vi "NI-Embedded CAN for RIO subVI - CAN Frame to Table1.vi"(6 "ramki":bool, 7 "Hexadecimal?":bool, 8 "error in (no error)":errorcluster, 9 "timestamp":timestamp, 10 "CAN frame":T1 {"type" items=["CAN Data", "CAN Remote"]; "identifier" format="%.0x"}, 11 "Input Array":string[][](array[string])) -> (0 "appended array":string[](array[string]), 1 "okres 1000":dbl, 3 "Output Array":string[][](array[string]), 4 "ilosc mesagy":dbl, 5 "okres 100":dbl)   [LabVIEW 2015]
doc: "This example shows how to put a CAN transceiver to sleep on RIO Embedded CAN devices."
uses:
  <vilib>/RioEmbeddedCAN/RioEmbeddedCAN.llb/CANFrameControl.ctl
panel:
  out "subarray 2":string[](array[string])
  out "subarray":string[](array[string])
  in  "Array":T1[](array[typedef]) {"type" items=["CAN Data", "CAN Remote"]; "identifier" format="%.0x"}
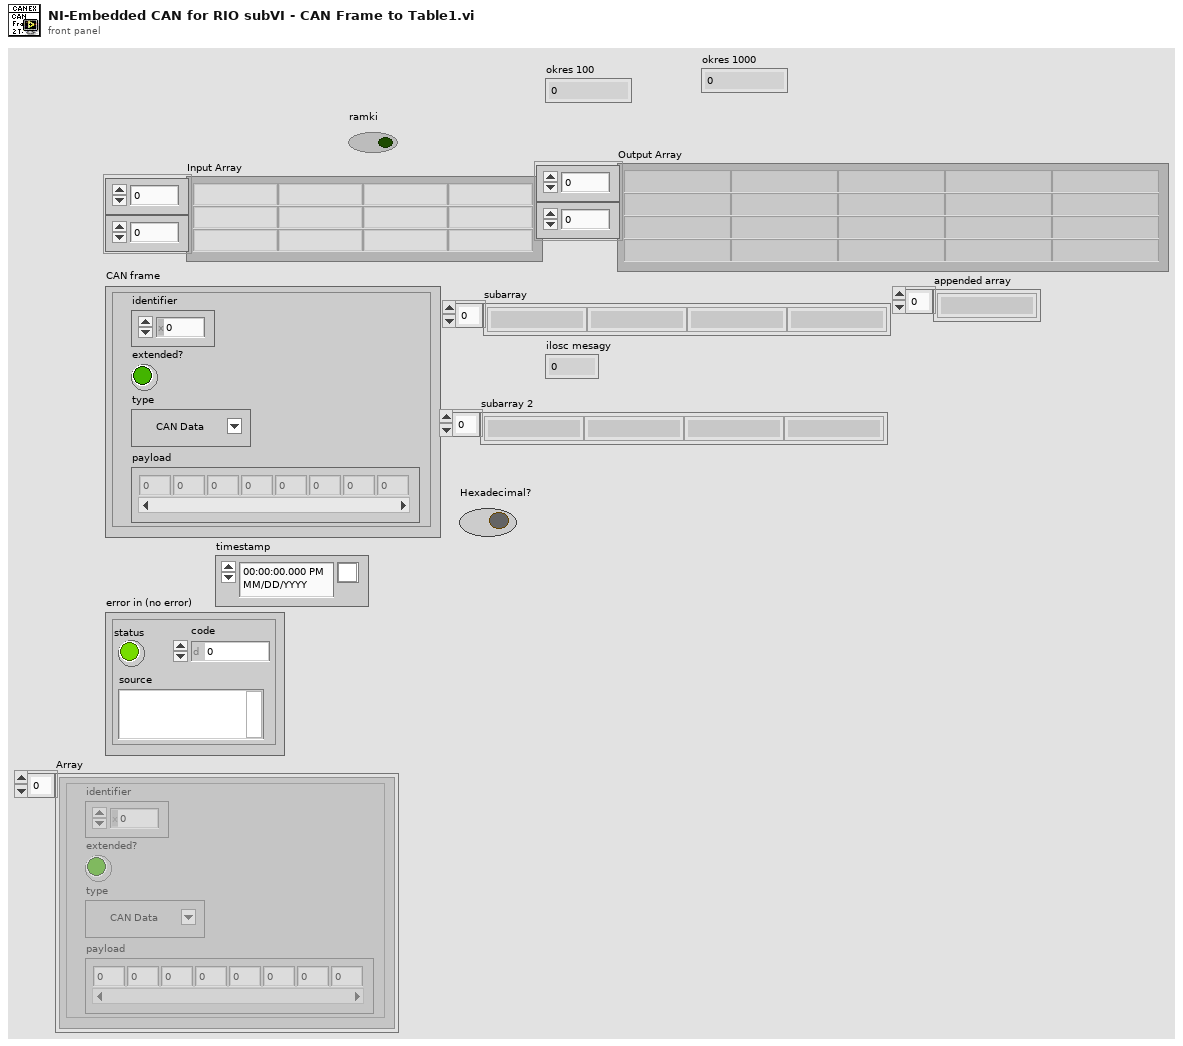
[diagram p1: front panel]
types:
  T1 = typedef "CANFrameControl.ctl" = cluster{"identifier":u32, "extended?":bool, "type":u8, "payload":u8[]}
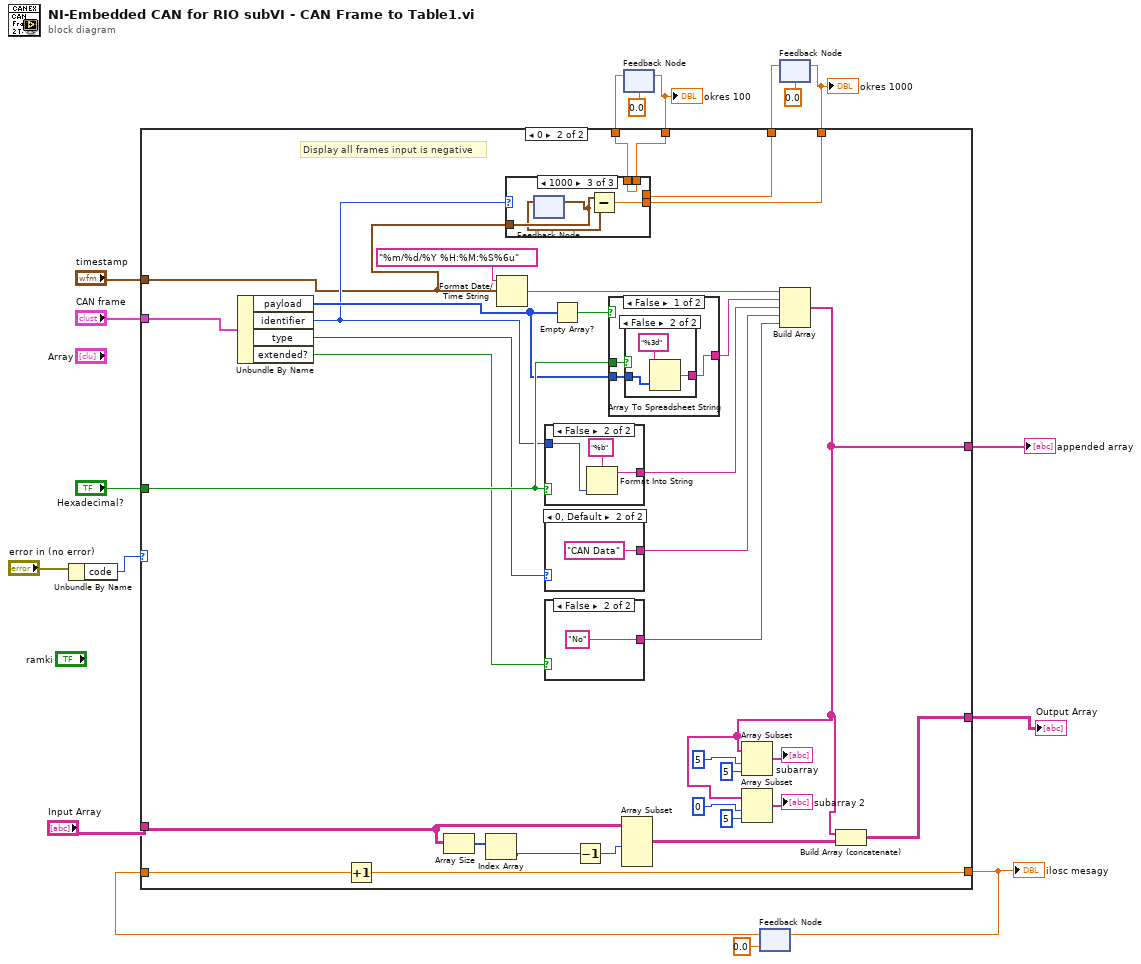
[diagram p0: block diagram]
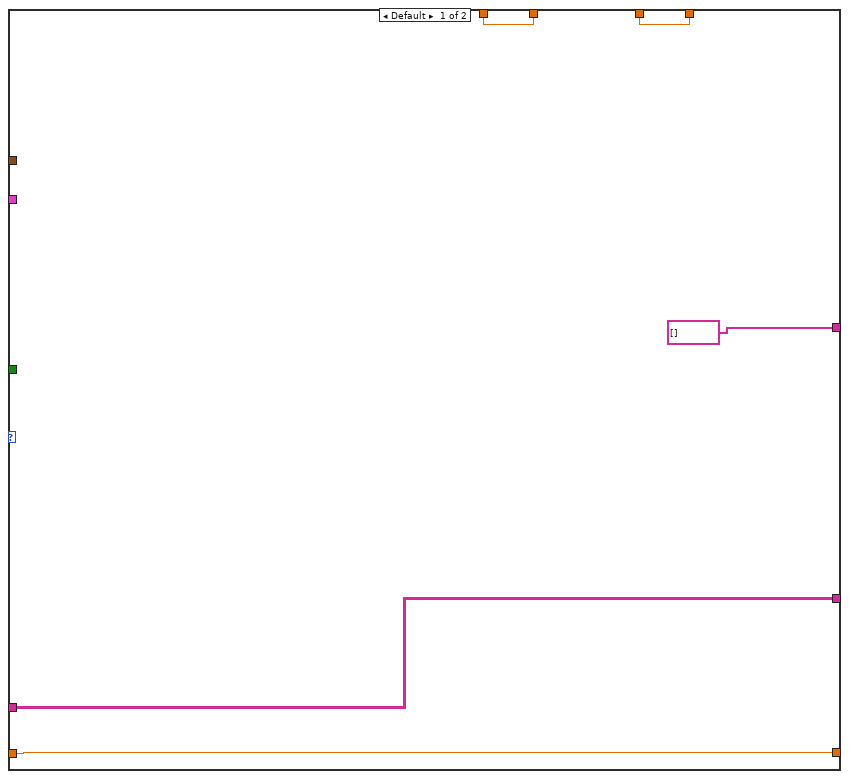
[diagram p2: hidden frame]
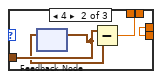
[diagram p4: hidden frame]
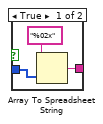
[diagram p5: hidden frame]
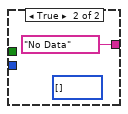
[diagram p6: hidden frame]
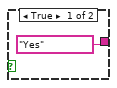
[diagram p7: hidden frame]
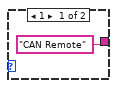
[diagram p8: hidden frame]
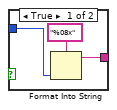
[diagram p9: hidden frame]
diagram:
  n1 = Unbundle By Name("error in (no error)") -> ("code"=w6:i32)
  n2 = feedback #1(0.0) -> (w4:dbl)
  n3 = feedback #2(0.0) -> (w10:dbl)
  n4 = feedback #3(0.0) -> (w3:dbl)
  n5 = case shown="0" w6 {
    tunnel: "Input Array" -> [w22 w54]
    tunnel: [w22 w53] -> w13
    tunnel: "Hexadecimal?" -> [_ w52]
    tunnel: "CAN frame" -> [_ w45]
    tunnel: "timestamp" -> [_ w27]
    tunnel: [w21 w47] -> w11
    tunnel: w10 -> [w21 w46]
    tunnel: [string[] [] w40] -> w12
    tunnel: [w19 w25] -> w5
    tunnel: w4 -> [w19 w23]
    tunnel: [w18 w26] -> w2
    tunnel: w3 -> [w18 w24]
    frame Default {
    }
    frame 0 {
      # "Display all frames input is negative"
      n6 = Unbundle By Name(w45) -> ("payload"=w30:u8[], "identifier"=w28:u32, "type"=w36:u8, "extended?"=w33:bool)
      n7 = Increment(x=w46) -> (x+1=w47:dbl)
      n8 = Array Size(array=w54) -> (size(s)=w55:i32[])
      n9 = Index Array(array=w55) -> (element=w41:i32)  [unwired: 1 in]
      n10 = Format Date/Time String(time format string (%c)="%m/%d/%Y %H:%M:%S%6u", seconds (now)=w27) -> (date/time string=w38:string)  [unwired: 1 in]
      n11 = case shown="1000" w28 {
        tunnel: w27 -> [_ w61 w65]
        tunnel: [w57 w58 w63] -> w26
        tunnel: [w56 w59 w62] -> w25
        tunnel: w24 -> [w57 w58 _]
        tunnel: w23 -> [w56 _ w62]
        frame 0, Default {
        }
        frame 4 {
          n12 = feedback #4() -> (w60:timestamp)  [unwired: 1 in]
          n13 = feedback-in #4(w61) -> ()
          n14 = Subtract(x=w61, y=w60) -> (x-y=w59:dbl)
        }
        frame 8 {
          n15 = feedback #5() -> (w64:timestamp)  [unwired: 1 in]
          n16 = feedback-in #5(w65) -> ()
          n17 = Subtract(x=w65, y=w64) -> (x-y=w63:dbl)
        }
      }
      n18 = case shown="False" w52 {
        tunnel: w28 -> [w81 w84]
        tunnel: [w80 w83] -> w37
        frame True {
          n19 = Format Into String(format string="%08x", w81) -> (resulting string=w80:string)  [unwired: 2 in, 1 out]
        }
        frame False {
          n20 = Format Into String(format string="%b", w84) -> (resulting string=w83:string)  [unwired: 2 in, 1 out]
        }
      }
      n21 = case shown="0, Default" w36 {
        tunnel: ["CAN Remote" "CAN Data"] -> w35
        frame 1 {
        }
        frame 0, Default {
        }
      }
      n22 = case shown="False" w33 {
        tunnel: ["Yes" "No"] -> w34
        frame True {
        }
        frame False {
        }
      }
      n23 = Empty Array?(array=w30) -> (empty?=w29:bool)
      n24 = Decrement(x=w41) -> (x-1=w42:i32)
      n25 = case shown="False" w29 {
        tunnel: [w66 "No Data"] -> w32
        tunnel: w30 -> [w68 _]
        tunnel: w52 -> [w67 _]
        frame False {
          n26 = case shown="False" w67 {
            tunnel: w68 -> [w69 w72]
            tunnel: [w70 w73] -> w66
            frame True {
              n27 = Array To Spreadsheet String(array=w69, 3:"%02x" ("format string")) -> (spreadsheet string=w70:string)  [unwired: 1 in]
            }
            frame False {
              n28 = Array To Spreadsheet String(array=w72, 3:"%3d" ("format string")) -> (spreadsheet string=w73:string)  [unwired: 1 in]
            }
          }
        }
        frame True {
          (unwired) u8[] [] ("payload")
        }
      }
      n29 = Array Subset(array=w54, length (row)=w42) -> (w39:string[][])  [unwired: 3 in]
      n30 = Build Array(w38, w32, w37, w35, w34) -> (w40:string[])
      n31 = Array Subset(array=w40, index=5 ("length"), length=5) -> (→"subarray":string[])
      n32 = Array Subset(array=w40, index=0 ("length"), length=5) -> (→"subarray 2":string[])
      n33 = Build Array (concatenate)(w40, w39) -> (w53:string[][])
    }
  }
  "Output Array" <- w13
  "ilosc mesagy" <- w11
  "appended array" <- w12
  "okres 100" <- w5
  "okres 1000" <- w2
  n34 = feedback-in #1(w5) -> ()
  n35 = feedback-in #2(w11) -> ()
  n36 = feedback-in #3(w2) -> ()
